vi "SetSyncDivider.vi"(11 "MH_UIThread_Data":T1 {"SyncDeadTime" min=800 max=160000 step=1; "SyncEdge" items=["falling", "rising"]; "SyncDivider" items=["1", "2", "4", "8", "16"]; "SyncOffset" min=0 max=100000 step=1; "SyncLevel" min=0 max=800 step=1; "AcqTime" min=1 max=360000 step=1; "Binning" items=["1", "2", "4", "8", "16", "32", "64", "128", "256", "512", "1024", "2048", "4096", "8192", "16384", "32768", "65536", "131072", "262144", "524288", "1048576", "2097152", "4194304", "8388608", "16777216", "3355443225"]; "HistoOffset" min=0 max=500 step=1; "HistoLen" min=1024 max=65536 step=1024; "Channels"."DeadTime" min=800 max=160000 step=1; "Channels"."Edge" items=["falling", "rising"]; "Channels"."Offset" min=-100000 max=100000 step=10; "Channels"."Level" min=-1200 max=1200 step=1}) -> (0 "error out":errorcluster)   [LabVIEW 2023]
uses:
  ConcreteClasses/ConcreteInstrumentClasses/Multiharp/Multiharp/Types/MH_InputChannel.ctl
  ConcreteClasses/ConcreteInstrumentClasses/Multiharp/Multiharp/Types/MH_SetInpChanCmds.ctl
  ConcreteClasses/ConcreteInstrumentClasses/Multiharp/Multiharp/Types/MH_SetInpChanData.ctl
  ConcreteClasses/ConcreteInstrumentClasses/Multiharp/Multiharp/Types/MH_UIThread_Data_T2.ctl
  ConcreteClasses/ConcreteInstrumentClasses/Multiharp/Multiharp/_lib/PQ/MultiHarp/MH_InitInfo.ctl
  typedefs/typedefs.lvlib
  <vilib>/ActorFramework/Message Enqueuer/Message Enqueuer.lvclass
panel:
  # "Sync"
  # "Histogram"
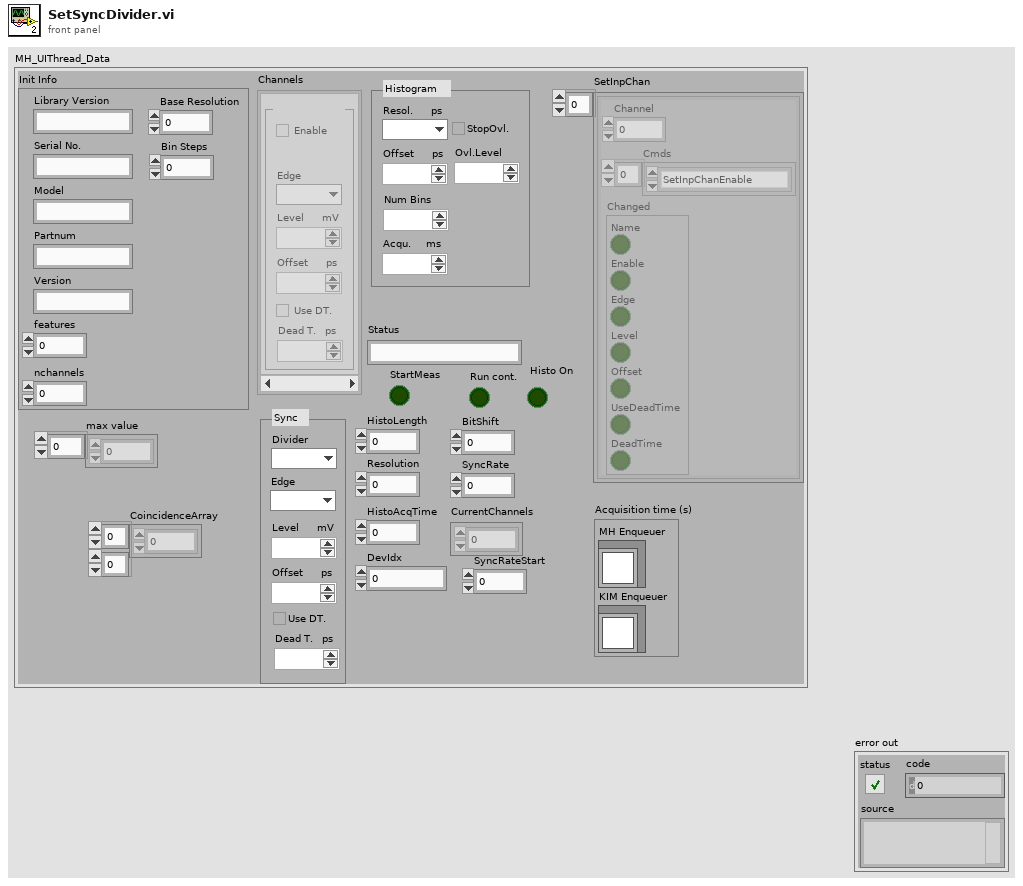
[diagram p1: front panel]
types:
  T1 = typedef "MH_UIThread_Data_T2.ctl" = cluster{"Init Info":T2, "DevIdx":i32, "SyncDivider":i32, "SyncOffset":i32, "SyncLevel":i32, "Channels":T3[], "CurrentChannels":i32[], "AcqTime":i32, "Binning":i32, "HistoOffset":i32, "HistoLen":i32, "StopOvl.":bool, "OvlLevel":u32, "SyncEdge":i32, "StartMeas":bool, "HistoLength":i32, "Resolution":dbl, "Run cont.":bool, "Status":string, "SyncRate":i32, "BitShift":i32, "HistoAcqTime":dbl, "SyncRateStart":i32, "UseDeadTime":bool, "SyncDeadTime":i32, "SetInpChan":T4[], "max value":u32[], "CoincidenceArray":dbl[][], "Instr Enqueuers":cluster{"MH Enqueuer":refnum<class "Message Enqueuer.lvclass">, "KIM Enqueuer":refnum<class "Message Enqueuer.lvclass">}, "Histo On":bool}
  T2 = typedef "typedefs.lvlib/MH_InitInfo.ctl" = cluster{"Library Version":string, "Serial No.":string, "Model":string, "Partnum":string, "Version":string, "features":i32, "nchannels":i32, "Base Resolution":dbl, "Bin Steps":i32}
  T3 = typedef "MH_InputChannel.ctl" = cluster{"Name":string, "Enable":bool, "Edge":i32, "Level":i32, "Offset":i32, "UseDeadTime":bool, "DeadTime":i32}
  T4 = typedef "MH_SetInpChanData.ctl" = cluster{"Channel":i32, "Cmds":T5[], "Changed":cluster{"Name":bool, "Enable":bool, "Edge":bool, "Level":bool, "Offset":bool, "UseDeadTime":bool, "DeadTime":bool}}
  T5 = typedef "MH_SetInpChanCmds.ctl" = enum16{"SetInpChanEnable", "SetInpChanOffset", "SetInpChanDeadTime", "SetInpChanTrg"}
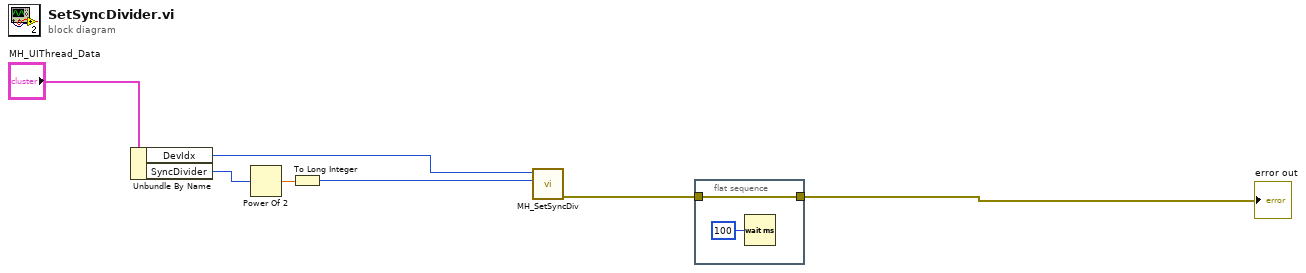
[diagram p0: block diagram]
diagram:
  n1 = Unbundle By Name("MH_UIThread_Data") -> ("DevIdx"=w2:i32, "SyncDivider"=w5:i32)
  n2 = Power Of 2(x=w5) -> (2^x=w6:dbl)
  n3 = To Long Integer(number=w6) -> (32bit integer=w7:i32)
  n4 = call "MH_SetSyncDiv.vi"("SyncDivider"=w7, "devidx"=w2) -> ("error out"=w3:errorcluster)  [unwired: 8 in, 1 out]
  n5 = flat-sequence {
    tunnel: w3 -> [w8]
    tunnel: [w8] -> w4
    frame #0 {
      n6 = Wait (ms)(milliseconds to wait=u32 100) -> ()  [unwired: 1 out]
    }
  }
  "error out" <- w4
